vi "Keithley6485 Bk.vi"(0 "Measure":refnum<vi>, 1 "Keithley6485 Online":refnum<vi>, 2 "Error In":refnum<vi>, 3 "Current (A)":refnum<vi>, 4 "Scan in Progress":refnum<vi>, 5 "Samples/Measurement":refnum<vi>, 7 "Perform Zero Correction":refnum<vi>, 8 "Enable Keithley6485":refnum<vi>, 9 "QUIT":refnum<vi>, 10 "Status":refnum<vi>, 11 "Keithley6485 picoAmmeter":refnum<visa-resource-name>="COM3") -> ()   [LabVIEW 2010]
uses:
  <vilib>/Utility/error.llb/DialogType.ctl
panel:
  out "Error Message":string=" INSTRUCTIONS:\r\rNormal Use:  When using subVIs that incorporate the error in/error out (or error I/O) structure, place this handler where you want to inform the user of an error, typically at the end of the I/O data path, as the last action of the program.  If the error in error? is ERROR, the handler creates a message describing the error and its source.  If the type of dialog = 1 (default), the message is displayed to the user, who can only acknowedge it.  If the type = 2, the user can acknowledge the message or abort execution; aborting a program with active I/O is not recommended.  If the type = 0, no message is displayed; this is used to process the error programmatically, and the error out cluster elements are wired to individual terminals for that reason.  \r\rOther Use:\n\r\nlocal testing.  To test the error code of a subVI or function that does not have the error I/O structure, you can wire its error code and a source string to the local error code and error source inputs.  If error in error? indicates no error and error code is not equal to 0, the local code and source are substituted for the error in values, and error? is set TRUE (ERROR)."
  in  "Timeout Extension Rate (ms/sample)":i32=500
  in  "Timeout Extension Offset (ms)":u32=1000
  # "Error out reports Serial I/O errors.\n\nKeithley Error reports error messages returned by the Keithley 6485 picoAmmeter.  Currently, only overvoltage and invalid data errors are supported by this VI."
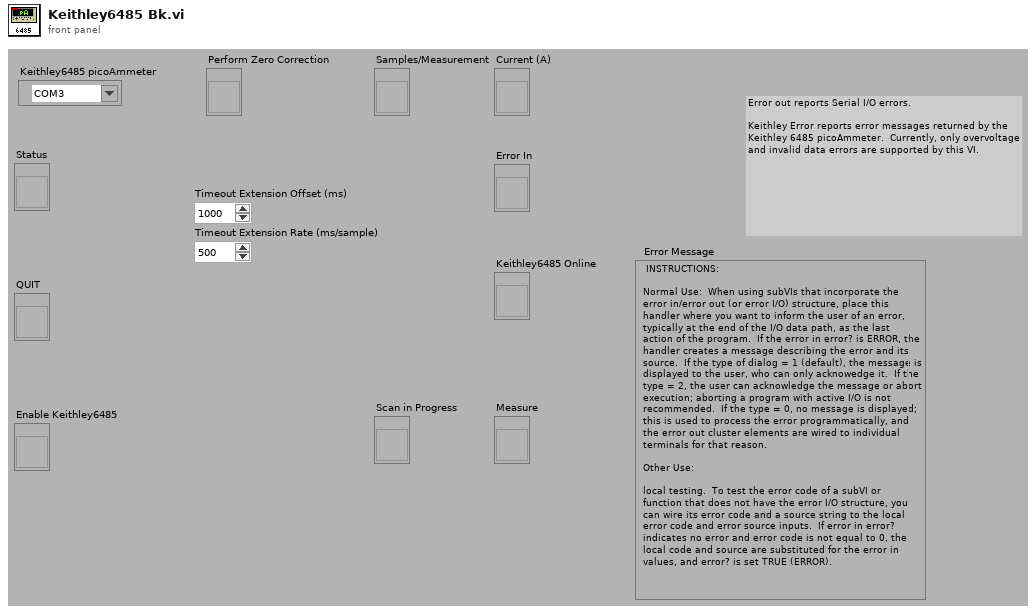
[diagram p1: front panel]
types:
  T1 = typedef "DialogType.ctl" = u16
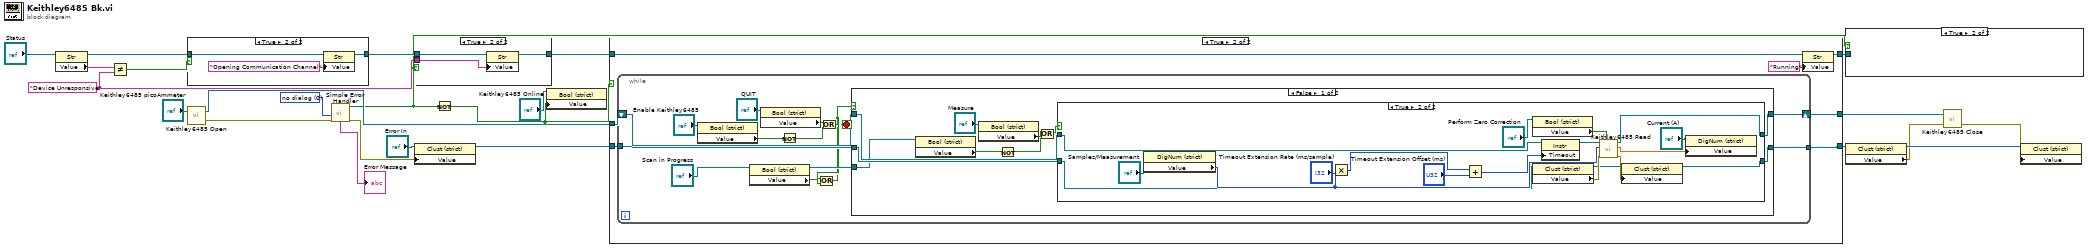
[diagram p0: block diagram]
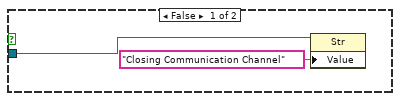
[diagram p3: hidden frame]
diagram:
  w4 = "Device Unresponsive" ("Value")
  w12 = T1 0 items=["no dialog", "OK message", "continue or stop message", "OK message + warnings", "continue/stop + warnings"] ("type of dialog (OK msg:1)")
  n1 = property on="Property Node" class="Str"(reference="Status") -> (reference out=w7:refnum<vi>, "Value"=w6:string)  [unwired: 1 in, 1 out]
  n2 = Not Equal?(x=w6, y=w4) -> (x != y?=w5:bool)
  n3 = case shown="True" w5 {
    tunnel: [w25 w28] -> w11
    tunnel: w7 -> [w25 w26]
    frame False {
    }
    frame True {
      n4 = property on="Property Node" class="Str"(reference=w26, "Value"="Opening Communication Channel") -> (reference out=w28:refnum<vi>)  [unwired: 1 in, 1 out]
    }
  }
  n5 = call "Keithley6485 Open.vi"("VISA resource name"="Keithley6485 picoAmmeter") -> ("Error out"=w15:errorcluster, "VISA out"=w16:refnum<visa-resource-name>)  [unwired: 1 in]
  n6 = call <vilib>:"Simple Error Handler.vi"("type of dialog (OK msg:1)"=w12, "error in (no error)"=w15) -> ("error?"=w9:bool, "error out"=w14:errorcluster, "message"=→"Error Message":string)  [unwired: 3 in, 2 out]
  n7 = case shown="True" w9 {
    tunnel: w11 -> [w29 w32]
    tunnel: [w29 w31] -> w10
    tunnel: w4 -> [_ w30]
    frame False {
    }
    frame True {
      n8 = property on="Property Node" class="Str"(reference=w32, "Value"=w30) -> (reference out=w31:refnum<vi>)  [unwired: 1 in, 1 out]
    }
  }
  n9 = property on="Property Node" class="Clust (strict)"(reference="Error In", "Value"=w14) -> (reference out=w3:refnum<vi>)  [unwired: 1 in, 1 out]
  n10 = Not(x=w9) -> (.not. x?=w22:bool)
  n11 = property on="Property Node" class="Bool (strict)"(reference="Keithley6485 Online", "Value"=w22) -> ()  [unwired: 1 in, 2 out]
  n12 = case shown="True" w22 {
    tunnel: w16 -> [w34 w42]
    tunnel: w10 -> [w35 w40]
    tunnel: [w34 w39] -> w18
    tunnel: [w35 w38] -> w17
    tunnel: w3 -> [w33 w37]
    tunnel: [w33 w36] -> w2
    frame False {
    }
    frame True {
      n13 = while {
        shift-right: [w55] -> w39
        shift-left: w42 -> [w56]
        tunnel: w37 -> [w49]
        tunnel: [w48] -> w36
        stop <- w43 stop-if-true
        n14 = property on="Property Node" class="Bool (strict)"(reference="Enable Keithley6485") -> ("Value"=w50:bool)  [unwired: 1 in, 2 out]
        n15 = property on="Property Node" class="Bool (strict)"(reference="Scan in Progress") -> (reference out=w46:refnum<vi>, "Value"=w45:bool)  [unwired: 1 in, 1 out]
        n16 = property on="Property Node" class="Bool (strict)"(reference="QUIT") -> ("Value"=w53:bool)  [unwired: 1 in, 2 out]
        n17 = Not(x=w50) -> (.not. x?=w51:bool)
        n18 = Or(x=w53, y=w51) -> (x .or. y?=w44:bool)
        n19 = Or(x=w44, y=w45) -> (x .or. y?=w43:bool)
        n20 = case shown="False" w44 {
          tunnel: w56 -> [w66 w88]
          tunnel: [w65 w88] -> w55
          tunnel: w49 -> [w64 w87]
          tunnel: [w63 w87] -> w48
          tunnel: w46 -> [w57 _]
          frame False {
            n21 = property on="Property Node" class="Bool (strict)"(reference=w57) -> ("Value"=w62:bool)  [unwired: 1 in, 2 out]
            n22 = property on="Property Node" class="Bool (strict)"(reference="Measure") -> ("Value"=w60:bool)  [unwired: 1 in, 2 out]
            n23 = Not(x=w62) -> (.not. x?=w59:bool)
            n24 = Or(x=w59, y=w60) -> (x .or. y?=w58:bool)
            n25 = case shown="True" w58 {
              tunnel: w66 -> [w68 w86]
              tunnel: [w68 w84] -> w65
              tunnel: w64 -> [w67 w70]
              tunnel: [w67 w69] -> w63
              frame False {
              }
              frame True {
                n26 = property on="Property Node" class="DigNum (strict)"(reference="Samples/Measurement") -> ("Value"=w71:i32)  [unwired: 1 in, 2 out]
                n27 = Multiply(x=w71, y="Timeout Extension Rate (ms/sample)") -> (x*y=w83:i32)
                n28 = Add(x=w83, y="Timeout Extension Offset (ms)") -> (x+y=w81:u32)
                n29 = property on="Property Node" class="Clust (strict)"(reference=w70) -> (reference out=w73:refnum<vi>, "Value"=w79:errorcluster)  [unwired: 1 in, 1 out]
                n30 = property on="Property Node" class="Bool (strict)"(reference="Perform Zero Correction") -> ("Value"=w77:bool)  [unwired: 1 in, 2 out]
                n31 = property class="Instr"(reference=w86, "Timeout"=w81) -> (reference out=w85:refnum<visa-resource-name>)  [unwired: 1 in, 1 out]
                n32 = call "Keithley6485 Read.vi"("Enable Zero Correction"=w77, "error in"=w79, "Sample per measurement"=w71, "VISA in"=w85) -> ("error out"=w78:errorcluster, "Current (A)"=w75:dbl, "VISA out"=w84:refnum<visa-resource-name>)  [unwired: 5 in]
                n33 = property on="Property Node" class="Clust (strict)"(reference=w73, "Value"=w78) -> (reference out=w69:refnum<vi>)  [unwired: 1 in, 1 out]
                n34 = property on="Property Node" class="DigNum (strict)"(reference="Current (A)", "Value"=w75) -> ()  [unwired: 1 in, 2 out]
              }
            }
          }
          frame True {
          }
        }
      }
      n35 = property on="Property Node" class="Str"(reference=w40, "Value"="Running") -> (reference out=w38:refnum<vi>)  [unwired: 1 in, 1 out]
    }
  }
  n36 = case shown="True" w9 {
    tunnel: w17 -> [w89 _]
    frame False {
      n37 = property on="Property Node" class="Str"(reference=w89, "Value"="Closing Communication Channel") -> ()  [unwired: 1 in, 2 out]
    }
    frame True {
    }
  }
  n38 = property on="Property Node" class="Clust (strict)"(reference=w2) -> (reference out=w20:refnum<vi>, "Value"=w19:errorcluster)  [unwired: 1 in, 1 out]
  n39 = call "Keithley6485 Close.vi"("error in"=w19, "VISA in"=w18) -> ("error out"=w21:errorcluster)  [unwired: 1 in]
  n40 = property on="Property Node" class="Clust (strict)"(reference=w20, "Value"=w21) -> ()  [unwired: 1 in, 2 out]
